vi "Append Value Length.vi"(8 "error in (no error)":errorcluster, 10 "Expect Value Length":i32, 11 "Plot Area Ref In":refnum<vi>) -> (0 "error out":errorcluster, 1 "Append Value?":bool, 2 "Actual Value Length":i32, 3 "Plot Area Ref Out":refnum<vi>)   [LabVIEW 2020, in "2D Plot.lvclass"]
uses:
  <vilib>/Math Plots/2D Math Plots/2D Plot/2D Plot/2D Plot.lvclass
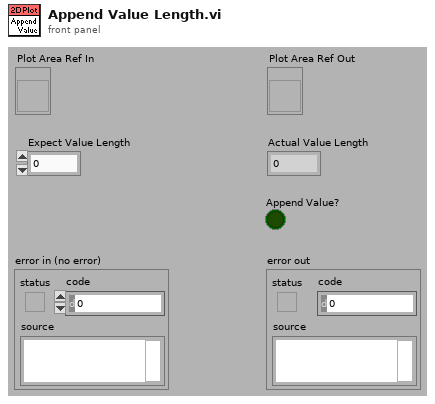
[diagram p1: front panel]
types:
  T1 = cluster{"Vertex X Array":dbl[], "Vertex Y Array":dbl[]}[]
  T2 = cluster{"Vertex X Array":dbl[], "Vertex Y Array":dbl[]}
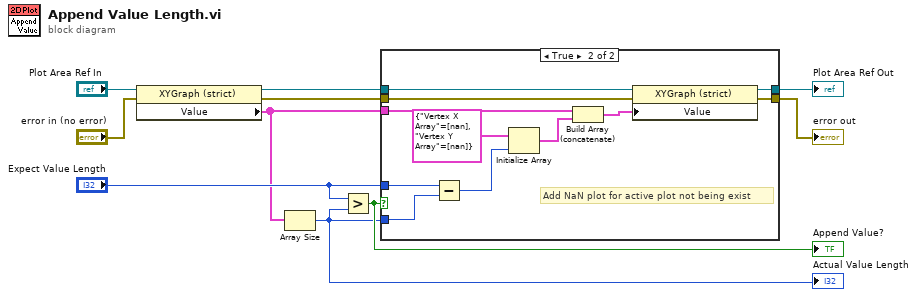
[diagram p0: block diagram]
diagram:
  n1 = property class="XYGraph (strict)"(reference="Plot Area Ref In", error in="error in (no error)") -> (reference out=w8:refnum<vi>, error out=w5:errorcluster, "Value"=w6:T1)
  n2 = Array Size(array=w6) -> (size(s)=w1:i32)
  "Actual Value Length" <- w1
  n3 = Greater?(x="Expect Value Length", y=w1) -> (0:w9:bool)
  "Append Value?" <- w9
  n4 = case shown="True" w9 {
    tunnel: w8 -> [w12 w23]
    tunnel: [w12 w22] -> w3
    tunnel: "Expect Value Length" -> [_ w21]
    tunnel: w1 -> [_ w20]
    tunnel: w6 -> [_ w17]
    tunnel: w5 -> [w11 w14]
    tunnel: [w11 w13] -> w2
    frame False {
    }
    frame True {
      # "Add NaN plot for active plot not being exist"
      n5 = Subtract(x=w21, y=w20) -> (x-y=w16:i32)
      n6 = Initialize Array(T2 {"Vertex X Array"=[nan], "Vertex Y Array"=[nan]} ("element"), w16) -> (w18:T1)
      n7 = Build Array (concatenate)(w17, w18) -> (w15:T1)
      n8 = property class="XYGraph (strict)"(reference=w23, error in=w14, "Value"=w15) -> (reference out=w22:refnum<vi>, error out=w13:errorcluster)
    }
  }
  "Plot Area Ref Out" <- w3
  "error out" <- w2
